vi "Write PositionIndex.vi"(8 "error in (no error)":errorcluster, 10 "Position":i32, 11 "OrderSelection in":refnum<class "OrderSelection.lvclass">) -> (0 "error out":errorcluster, 3 "OrderSelection out":refnum<class "OrderSelection.lvclass">)   [LabVIEW 2015, in "OrderSelection.lvclass"]
uses:
  OrderSelection.lvclass
  OrderSelection.lvclass/OrderSelection.ctl
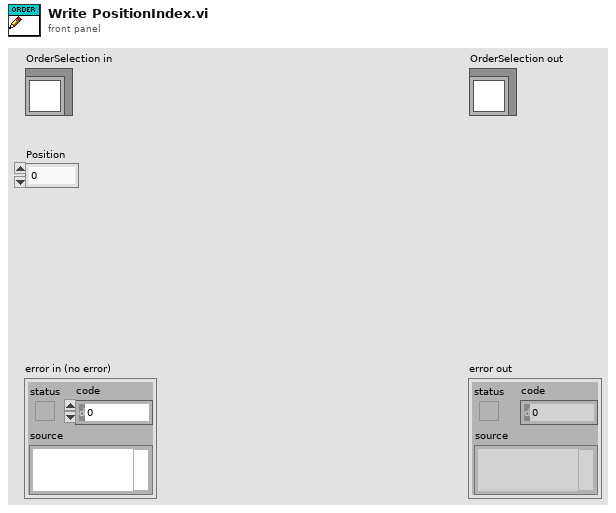
[diagram p1: front panel]
types:
  T1 = typedef "OrderSelection.lvclass/State Data.ctl" = cluster{"Items[]":string[], "SelectedItem":i32, "Position":i32, "ItemGraphic":T2}
  T2 = typedef "imagedata.ctl" = cluster{"image type":i32, "image depth":i32, "image":u8[], "mask":u8[], "colors":u32[], "Rectangle":cluster{"left":i16, "top":i16, "right":i16, "bottom":i16}}
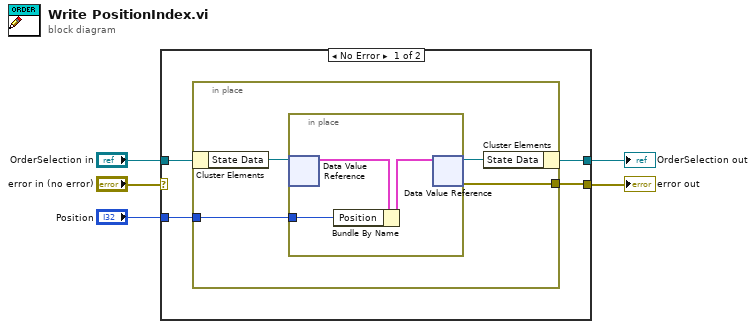
[diagram p0: block diagram]
diagram:
  n1 = case shown="No Error" "error in (no error)" {
    selector: "error in (no error)" -> [_ w18]
    tunnel: [w6 w18] -> w4
    tunnel: [w7 w17] -> w2
    tunnel: "OrderSelection in" -> [w9 w17]
    tunnel: "Position" -> [w8 _]
    frame No Error {
      n2 = in-place {
        in-place-border: w8 -> [w12]
        in-place-border: [w10] -> w6
        n3 = in-place-cluster #1(w9) -> ("State Data"=w13:refnum<data-value>)
        n4 = in-place {
          in-place-border: w12 -> [w15]
          n5 = in-place-dvr #2(w13) -> (w16:T1)  [unwired: 1 out]
          n6 = Bundle By Name(cluster=w16, "Position"=w15) -> (w14:T1)
          n7 = in-place-dvr #2(w14) -> (w11:refnum<data-value>, w10:errorcluster)
        }
        n8 = in-place-cluster #1("State Data"=w11) -> (w7:refnum<class "OrderSelection.lvclass">)
      }
    }
    frame Error {
    }
  }
  "error out" <- w4
  "OrderSelection out" <- w2
